vi "f_create file and save data.vi"(7 "operation (0:open)":T1(ring), 8 "1D data":dbl[](array[numeric]), 9 "2D data":dbl[][](array[numeric]), 10 "path":path) -> (0 "error out":errorcluster)   [LabVIEW 2016]
uses:
  <vilib>/Utility/file.llb/Write Delimited Spreadsheet (DBL).vi
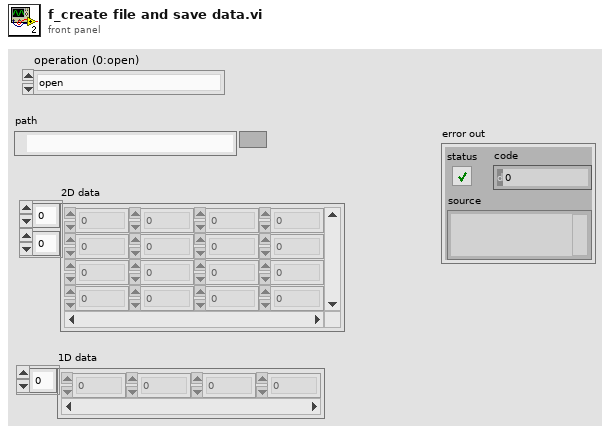
[diagram p1: front panel]
types:
  T1 = enum16{"open", "replace", "create", "open or create", "replace or create", "replace or create with confirmation"}
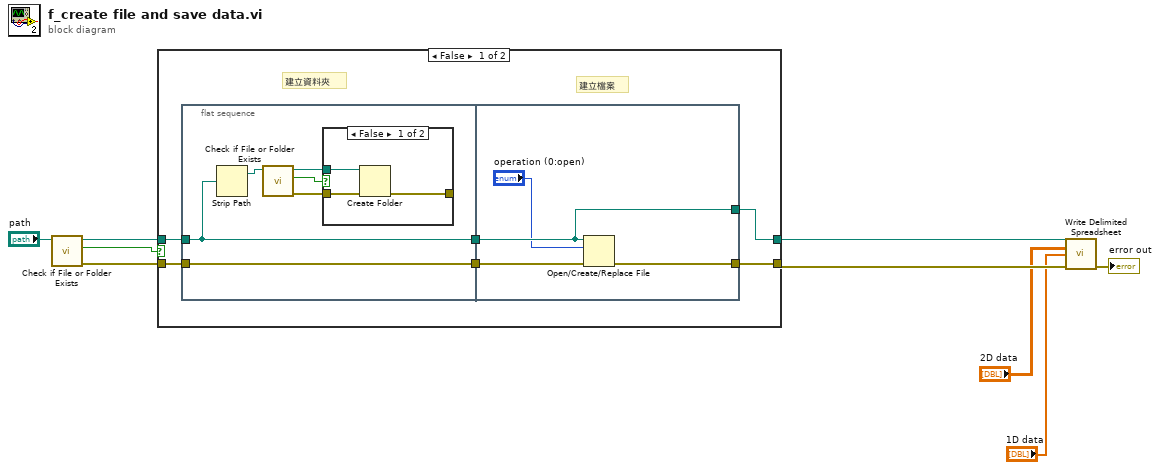
[diagram p0: block diagram]
diagram:
  n1 = call <vilib>:"Check if File or Folder Exists.vi"("path"="path") -> ("error out"=w6:errorcluster, "file or folder exists?"=w8:bool, "dup path"=w7:path)  [unwired: 8 in]
  n2 = case shown="False" w8 {
    tunnel: w7 -> [w14 w31]
    tunnel: w6 -> [w15 w30]
    tunnel: [w13 w30] -> w5
    tunnel: [w12 w31] -> w3
    frame False {
      # "建立檔案"
      # "建立資料夾"
      n3 = flat-sequence {
        tunnel: w14 -> [w16]
        tunnel: w15 -> [w21]
        tunnel: [w21] -> w11
        tunnel: [w16] -> w10
        tunnel: [w28] -> w13
        tunnel: [w27] -> w12
        tunnel: w11 -> [w29]
        tunnel: w10 -> [w27]
        frame #0 {
          n4 = Strip Path(path=w16) -> (stripped path=w17:path)  [unwired: 1 out]
          n5 = call <vilib>:"Check if File or Folder Exists.vi"("path"=w17) -> ("error out"=w20:errorcluster, "file or folder exists?"=w18:bool, "dup path"=w19:path)  [unwired: 8 in]
          n6 = case shown="False" w18 {
            tunnel: w19 -> [w24 _]
            tunnel: [w23 w25] -> _
            tunnel: w20 -> [w22 w25]
            frame False {
              n7 = Create Folder(path (use dialog)=w24, error in=w22) -> (error out=w23:errorcluster)  [unwired: 1 in, 2 out]
            }
            frame True {
            }
          }
        }
        frame #1 {
          n8 = Open/Create/Replace File(file path (use dialog)=w27, error in=w29, operation (0:open)="operation (0:open)") -> (error out=w28:errorcluster)  [unwired: 3 in, 2 out]
        }
      }
    }
    frame True {
    }
  }
  n9 = call-poly <vilib>:"Write Delimited Spreadsheet.vi"("file path (dialog if empty)"=w3, "2D data"="2D data", "1D data"="1D data", "error in (no error)"=w5) -> ("error out"=→"error out":errorcluster)  [unwired: 10 in, 1 out]
